vi "Sample.vi"() -> ()   [LabVIEW 2013]
uses:
  <vilib>/Utility/error.llb/DialogType.ctl
  Data/ReadVoltageSetting(General).vi
  Data/ReadCurrentSetting(General).vi
  Data/ReadFrequencySetting(General).vi
  Data/ReadPowerSetting(General).vi
  Configure/SetVoltage(General).vi
  Configure/SetCurrent(General).vi
  Configure/SetFrequency(General).vi
  Configure/SetPower(General).vi
panel:
  out "General Setting Change":bool
  in  "General Settings":T1={"Voltage"=0.0, "A-Hi Limit"=0.0, "Frequency"=15.0, "P-Hi Limit"=0} {"P-Hi Limit" max=500 step=1 format="%.0f W"; "A-Hi Limit" min=0.0 max=5.0 step=1.0 format="%.2f A"; "Frequency" min=15.0 max=1000.0 step=1.0 format="%.1f Hz"; "Voltage" min=0.0 max=310.0 step=1.0 format="%.1f V"}
  out "Real-Time Meter":T2 {"Power" format="%.0f W"; "Current" format="%.2f A"; "Frequency" format="%.1f Hz"; "Voltage" format="%.1f V"}
  in  "stop":bool
  in  "RESET":bool
  in  "OUTPUT":bool
  in  "VISA resource name":refnum<visa-resource-name>
  in  "baud rate (115200)":u32=115200
  # "Channel Settings"
  # "OUTPUT\nControl"
  # "Real-Time Meter"
  # "General Settings"
  # "Stop VI"
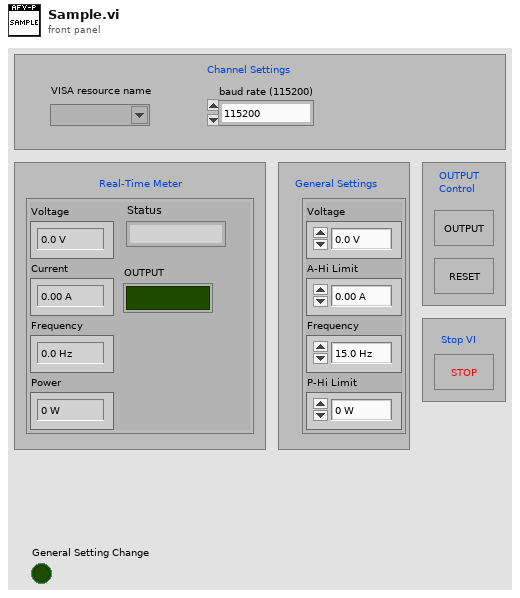
[diagram p1: front panel]
types:
  T1 = cluster{"Voltage":dbl, "A-Hi Limit":dbl, "Frequency":dbl, "P-Hi Limit":u16}
  T2 = cluster{"Voltage":dbl, "Current":dbl, "Frequency":dbl, "Power":dbl, "Status":string, "OUTPUT":bool}
  T3 = typedef "DialogType.ctl" = u16
  T4 = cluster{"Setting":dbl, "Setting":dbl, "Setting":dbl, "Setting":dbl}
  T5 = cluster{"Mode":string, "AC/DC":string, "Memory":dbl, "Step":dbl, "States":string, "Time Unit":string, "V":dbl, "A":dbl, "F":dbl, "P":dbl, "VA":dbl, "CF":dbl, "Ap":dbl, "Q":dbl, "PF":dbl, "T":dbl}
  T6 = cluster{"V":dbl, "A":dbl, "F":dbl, "P":dbl, "States":string, "ON/OFF":bool}
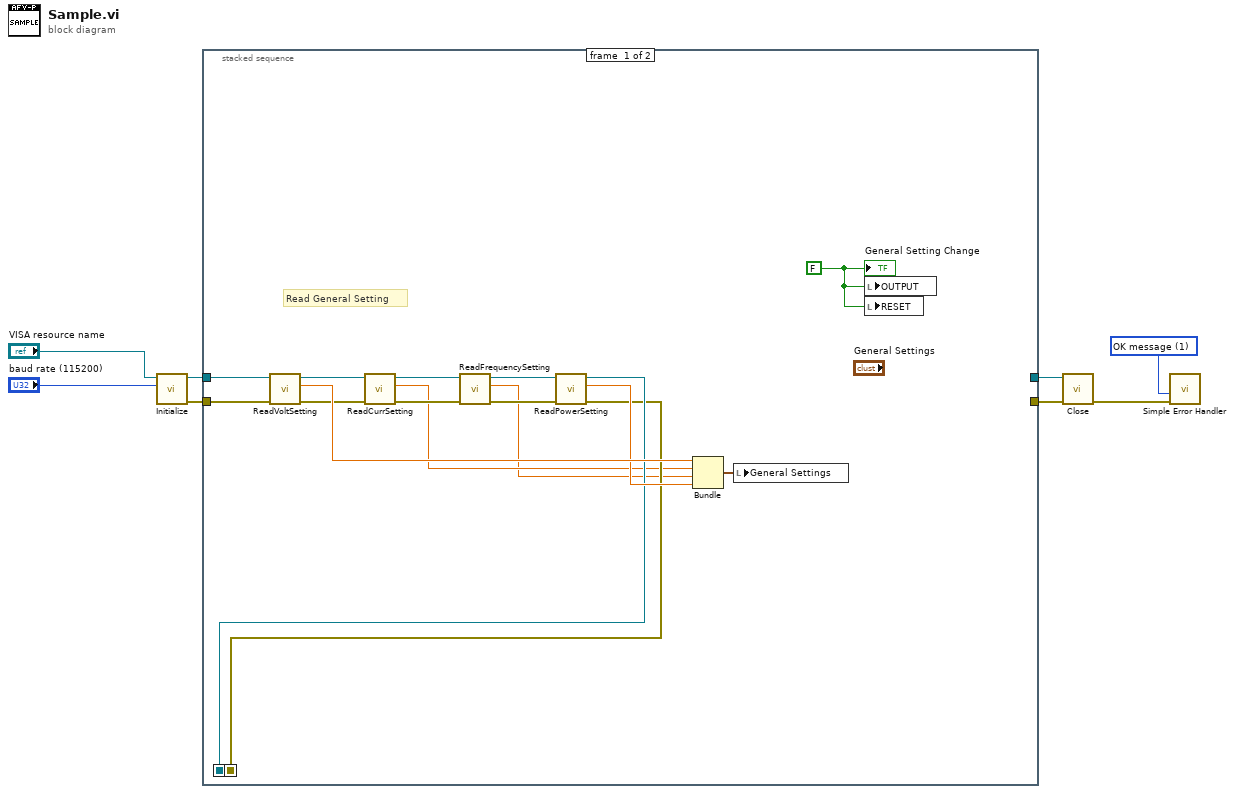
[diagram p0: block diagram]
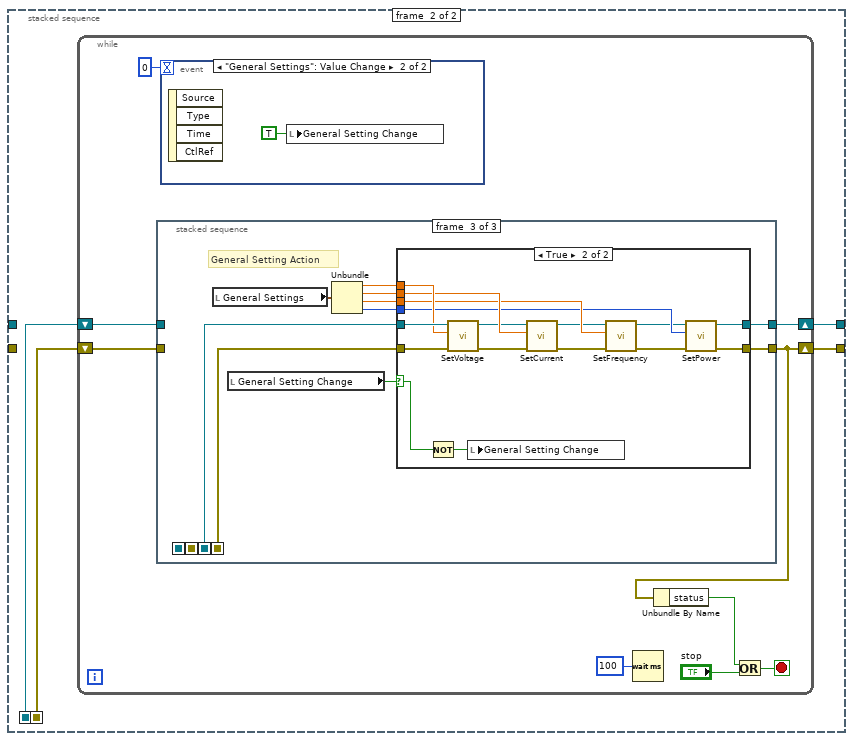
[diagram p2: hidden frame]
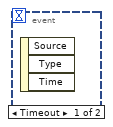
[diagram p3: hidden frame]
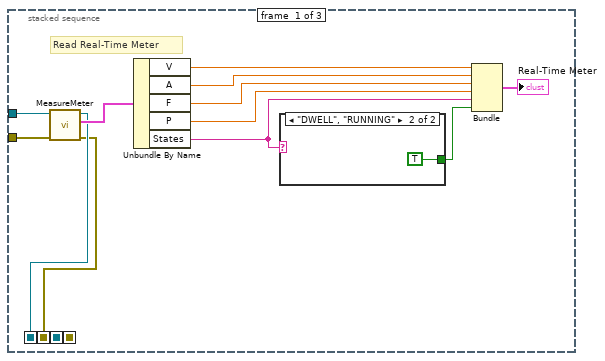
[diagram p4: hidden frame]
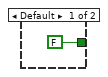
[diagram p5: hidden frame]
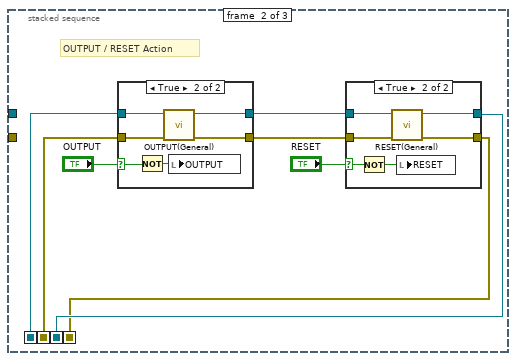
[diagram p6: hidden frame]
diagram:
  w1 = T3 1 items=["no dialog", "OK message", "continue or stop message", "OK message + warnings", "continue/stop + warnings"] ("type of dialog (OK msg:1)")
  n1 = call "Initialize.vi"("baud rate (115200)"="baud rate (115200)", "VISA resource name"="VISA resource name") -> ("error out"=w5:errorcluster, "VISA resource name out"=w6:refnum<visa-resource-name>)  [unwired: 8 in]
  n2 = stacked-sequence {
    seq-local: [w18 _] -> [_ w28]
    seq-local: [w17 _] -> [_ w27]
    tunnel: w6 -> [w22 _]
    tunnel: w5 -> [w21 _]
    tunnel: [_ w26] -> w4
    tunnel: [_ w25] -> w3
    frame #0 {
      w23 = FALSE ("General Setting Change")
      # "Read General Setting"
      n3 = call-poly "ReadVoltSetting.vi"("Error In"=w21, "VISA resource name"=w22) -> ("Error Out"=w12:errorcluster, "Setting"=w20:dbl, "VISA resource name out"=w16:refnum<visa-resource-name>)  [unwired: 7 in]
      n4 = call-poly "ReadCurrSetting.vi"("Error In"=w12, "VISA resource name"=w16) -> ("Error Out"=w11:errorcluster, "Setting"=w10:dbl, "VISA resource name out"=w15:refnum<visa-resource-name>)  [unwired: 7 in]
      n5 = call-poly "ReadFrequencySetting.vi"("Error In"=w11, "VISA resource name"=w15) -> ("Error Out"=w13:errorcluster, "Setting"=w9:dbl, "VISA resource name out"=w14:refnum<visa-resource-name>)  [unwired: 7 in]
      n6 = call-poly "ReadPowerSetting.vi"("Error In"=w13, "VISA resource name"=w14) -> ("Error Out"=w17:errorcluster, "Setting"=w19:dbl, "VISA resource name out"=w18:refnum<visa-resource-name>)  [unwired: 7 in]
      n7 = Bundle("Setting"=w20, "Setting"=w10, "Setting"=w9, "Setting"=w19) -> (w24:T4)  [unwired: 1 in]
      n8 = local write "General Settings"(w24) -> ()
      n9 = local write "OUTPUT"(w23) -> ()
      n10 = local write "RESET"(w23) -> ()
      "General Setting Change" <- w23
    }
    frame #1 {
      n11 = while {
        shift-right: [w34] -> w26
        shift-left: w28 -> [w36]
        shift-right: [w32] -> w25
        shift-left: w27 -> [w35]
        stop <- w31 stop-if-true
        n12 = stacked-sequence {
          seq-local: [w45 _ _] -> [_ w58 _]
          seq-local: [w44 _ _] -> [_ w57 _]
          seq-local: [_ w54 _] -> [_ _ w82]
          seq-local: [_ w53 _] -> [_ _ w83]
          tunnel: w36 -> [w43 _ _]
          tunnel: w35 -> [w42 _ _]
          tunnel: [_ _ w85] -> w34
          tunnel: [_ _ w84] -> w32
          frame #0 {
            # "Read Real-Time Meter"
            n13 = call "MeasureMeter.vi"("Error In"=w42, "VISA resource name"=w43) -> ("Error Out"=w44:errorcluster, "Meter"=w50:T5, "VISA resource name out"=w45:refnum<visa-resource-name>)  [unwired: 7 in]
            n14 = Unbundle By Name(w50) -> ("V"=w49:dbl, "A"=w48:dbl, "F"=w47:dbl, "P"=w46:dbl, "States"=w40:string)
            n15 = case shown="\"DWELL\", \"RUNNING\"" w40 {
              tunnel: [FALSE ("ON/OFF") TRUE ("ON/OFF")] -> w41
              frame Default {
              }
              frame "DWELL", "RUNNING" {
              }
            }
            n16 = Bundle("V"=w49, "A"=w48, "F"=w47, "P"=w46, "States"=w40, "ON/OFF"=w41) -> (→"Real-Time Meter":T6)  [unwired: 1 in]
          }
          frame #1 {
            # "OUTPUT / RESET Action"
            n17 = case shown="True" "OUTPUT" {
              selector: "OUTPUT" -> [_ w72]
              tunnel: w58 -> [w70 w76]
              tunnel: w57 -> [w69 w75]
              tunnel: [w70 w74] -> w56
              tunnel: [w69 w73] -> w55
              frame False {
              }
              frame True {
                n18 = Not(x=w72) -> (.not. x?=w71:bool)
                n19 = call "OUTPUT(General).vi"("Error In"=w75, "VISA resource name"=w76) -> ("Error Out"=w73:errorcluster, "VISA resource name out"=w74:refnum<visa-resource-name>)  [unwired: 8 in]
                n20 = local write "OUTPUT"(w71) -> ()
              }
            }
            n21 = case shown="True" "RESET" {
              selector: "RESET" -> [_ w63]
              tunnel: w56 -> [w62 w68]
              tunnel: w55 -> [w61 w67]
              tunnel: [w62 w66] -> w54
              tunnel: [w61 w65] -> w53
              frame False {
              }
              frame True {
                n22 = Not(x=w63) -> (.not. x?=w64:bool)
                n23 = call "RESET(General).vi"("Error In"=w67, "VISA resource name"=w68) -> ("Error Out"=w65:errorcluster, "VISA resource name out"=w66:refnum<visa-resource-name>)  [unwired: 8 in]
                n24 = local write "RESET"(w64) -> ()
              }
            }
          }
          frame #2 {
            # "General Setting Action"
            n25 = local read "General Settings"() -> (w81:T1)
            n26 = local read "General Setting Change"() -> (w86:bool)
            n27 = Unbundle(w81) -> ("Voltage"=w80:dbl, "A-Hi Limit"=w79:dbl, "Frequency"=w78:dbl, "P-Hi Limit"=w77:u16)
            n28 = case shown="True" w86 {
              selector: w86 -> [_ w103]
              tunnel: w83 -> [w87 w101]
              tunnel: w82 -> [w88 w102]
              tunnel: [w88 w90] -> w85
              tunnel: [w87 w89] -> w84
              tunnel: w80 -> [_ w100]
              tunnel: w79 -> [_ w99]
              tunnel: w78 -> [_ w98]
              tunnel: w77 -> [_ w97]
              frame False {
              }
              frame True {
                n29 = Not(x=w103) -> (.not. x?=w104:bool)
                n30 = call-poly "SetVoltage.vi"("Error In"=w101, "Voltage"=w100, "VISA resource name"=w102) -> ("Error Out"=w93:errorcluster, "VISA resource name out"=w94:refnum<visa-resource-name>)  [unwired: 7 in]
                n31 = local write "General Setting Change"(w104) -> ()
                n32 = call-poly "SetCurrent.vi"("Error In"=w93, "Current"=w99, "VISA resource name"=w94) -> ("Error Out"=w92:errorcluster, "VISA resource name out"=w95:refnum<visa-resource-name>)  [unwired: 7 in]
                n33 = call-poly "SetFrequency.vi"("Error In"=w92, "Frequency"=w98, "VISA resource name"=w95) -> ("Error Out"=w91:errorcluster, "VISA resource name out"=w96:refnum<visa-resource-name>)  [unwired: 7 in]
                n34 = call-poly "SetPower.vi"("Error In"=w91, "Power"=w97, "VISA resource name"=w96) -> ("Error Out"=w89:errorcluster, "VISA resource name out"=w90:refnum<visa-resource-name>)  [unwired: 7 in]
              }
            }
          }
        }
        n35 = event shown="[1] \"General Settings\": Value Change" {
          selector: _ -> [_ _]
          dyn-events: _ -> [_ _]
          timeout: 0 -> [_ _]
          event Timeout {
            n36 = event-data() -> ()  [unwired: 1 in, 3 out]
          }
          event "General Settings": Value Change {
            n37 = event-data() -> ()  [unwired: 1 in, 4 out]
            n38 = local write "General Setting Change"(TRUE ("General Setting Change")) -> ()
          }
        }
        n39 = Wait (ms)(milliseconds to wait=u32 100) -> ()  [unwired: 1 out]
        n40 = Unbundle By Name(w32) -> ("status"=w29:bool)
        n41 = Or(x=w29, y="stop") -> (x .or. y?=w31:bool)
      }
    }
  }
  n42 = call "Close.vi"("error in"=w3, "VISA resource name"=w4) -> ("error out"=w2:errorcluster)  [unwired: 9 in]
  n43 = call <vilib>:"Simple Error Handler.vi"("type of dialog (OK msg:1)"=w1, "error in (no error)"=w2) -> ()  [unwired: 3 in, 5 out]
